vi "MatrixReset.vi"(8 "error in (no error)":errorcluster, 11 "Pickering in":refnum<class "PickeringPrague.lvclass">) -> (0 "error out":errorcluster, 3 "Pickering out":refnum<class "PickeringPrague.lvclass">)   [LabVIEW 2018, in "PickeringPrague.lvclass"]
uses:
  PickeringPrague.lvclass
  C:/Users/itk/Documents/itk-strip-sensor-qc/InstrControl/InstrControl.lvclass
  PickeringMatrix_CommandsGlobal.vi
  InstrControl.lvclass
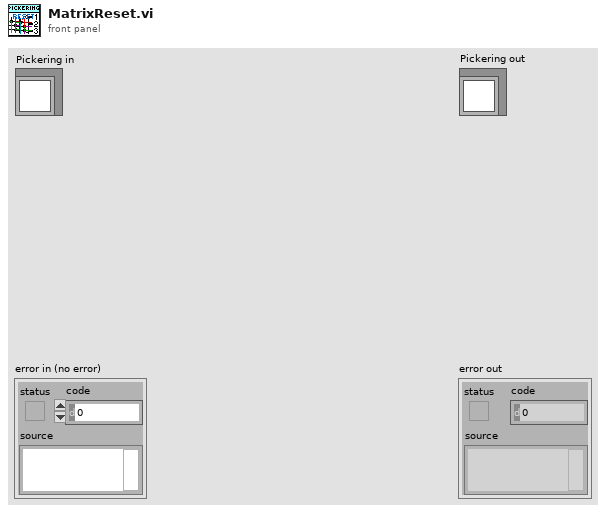
[diagram p1: front panel]
types:
  T1 = cluster{"Matrix address":string, "Instrument name":string, "Instrument type":u16, "Command \"Matrix Reset\"":string, "Command \"Connect Matrix Channels\"":string, "Command \"Disconnect Matrix Channels\"":string}
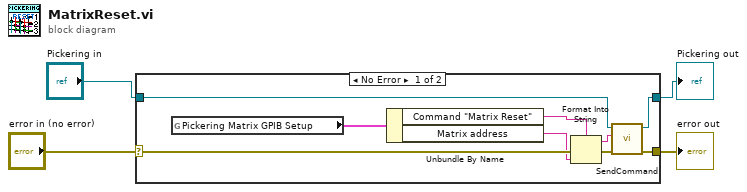
[diagram p0: block diagram]
diagram:
  n1 = case shown="No Error" "error in (no error)" {
    selector: "error in (no error)" -> [w11 w15]
    tunnel: [w6 w15] -> w1
    tunnel: [w12 w14] -> w2
    tunnel: "Pickering in" -> [w13 w14]
    frame No Error {
      n2 = global read "PickeringMatrix_CommandsGlobal.vi" "Pickering Matrix GPIB Setup"() -> (w5:T1)
      n3 = Unbundle By Name(w5) -> ("Command \"Matrix Reset\""=w9:string, "Matrix address"=w10:string)
      n4 = Format Into String(format string=w9, error in=w11, w10) -> (resulting string=w8:string, error out=w7:errorcluster)  [unwired: 1 in]
      n5 = call "SendCommand.vi"("error in (no error)"=w7, "Command string"=w8, "InstControl in"=w13) -> ("error out"=w6:errorcluster, "InstControl out"=w12:refnum<class "PickeringPrague.lvclass">)  [unwired: 7 in]
    }
    frame Error {
    }
  }
  "error out" <- w1
  "Pickering out" <- w2
